vi "ccd_imaging.vi"() -> ()   [LabVIEW 2009]
panel:
  in  "File path: manual (up) or automatic (down)?":bool
  in  "Or, read path automatically from:":path=path "\\\\Foghorn.bio.brandeis.edu\\remote"
  in  "Manual save directory":string
  in  "Manual save path":path
  in  "Triggered scanning":bool
  in  "Live scan / snapshots":bool
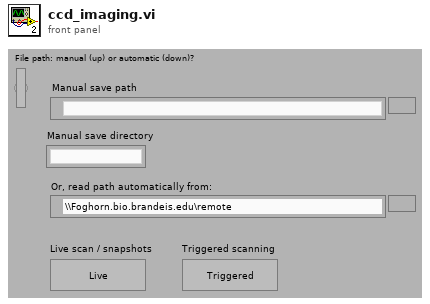
[diagram p1: front panel]
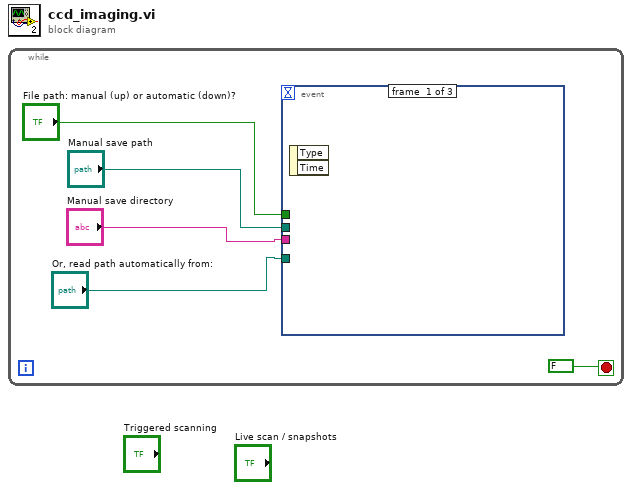
[diagram p0: block diagram]
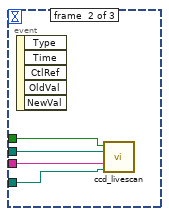
[diagram p2: hidden frame]
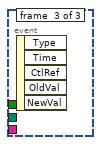
[diagram p3: hidden frame]
diagram:
  n1 = while {
    stop <- FALSE stop-if-true
    n2 = event shown="[1] \"Live scan / snapshots\": Value Change" {
      selector: _ -> [_ _ _]
      dyn-events: _ -> [_ _ _]
      timeout: _ -> [_ _ _]
      tunnel: "File path: manual (up) or automatic (down)?" -> [_ w9 _]
      tunnel: "Manual save path" -> [_ w8 _]
      tunnel: "Manual save directory" -> [_ w7 _]
      tunnel: "Or, read path automatically from:" -> [_ w6 _]
      event #0 {
        n3 = event-data() -> ()  [unwired: 1 in, 2 out]
      }
      event #1 {
        n4 = event-data() -> ()  [unwired: 1 in, 5 out]
        n5 = call "ccd_livescan.vi"("Or, read path automatically from:"=w6, "Manual save directory"=w7, "Manual save path"=w8, "Manual (up) or automatic (down)"=w9) -> ()  [unwired: 8 in]
      }
      event #2 {
        n6 = event-data() -> ()  [unwired: 1 in, 5 out]
      }
    }
  }
